vi "Jog.vi"(0 "AXIS Array":i32[](array[numeric]), 1 "U":bool, 2 "D":bool, 3 "R":bool, 4 "L":bool, 6 "Jog_Speed":i32=10000, 7 "Jog_相對位置":dbl format="%.2f", 9 "相對位置移動":bool, 10 "Jog Ring":u16(ring) items=["Step", "Continuous"], 11 "Step Ring":u16(ring) items=["0.001 mm", "0.01 mm", "0.1 mm", "1 mm"]) -> ()   [LabVIEW 2015]
uses:
  <userlib>/ADLINK/APS168.lvlib
panel:
  in  "角度逆轉":bool
  in  "角度正轉":bool
  in  "正轉":bool
  in  "逆轉":bool
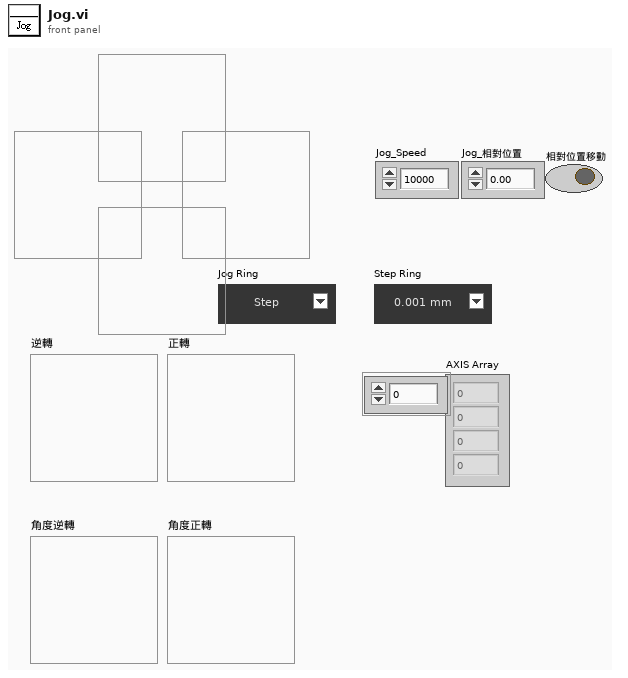
[diagram p1: front panel]
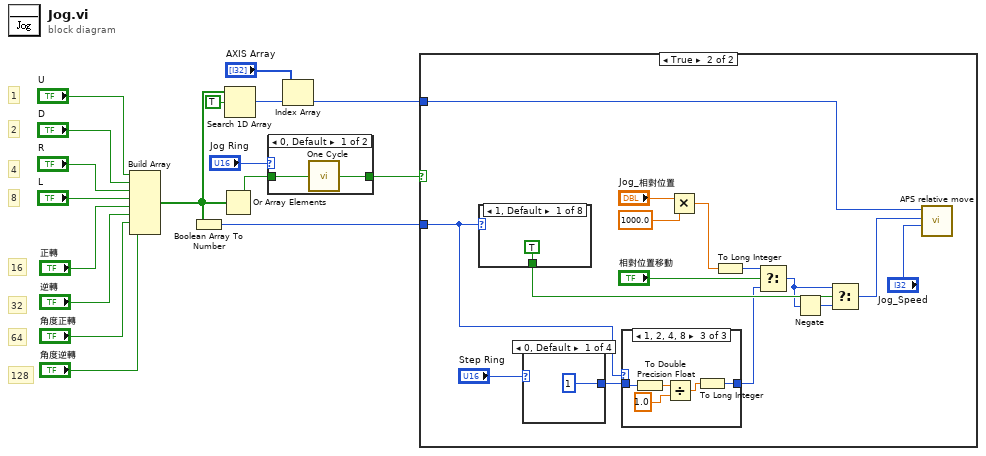
[diagram p0: block diagram]
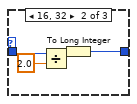
[diagram p5: hidden frame]
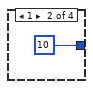
[diagram p6: hidden frame]
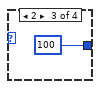
[diagram p7: hidden frame]
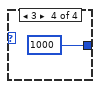
[diagram p8: hidden frame]
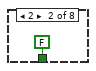
[diagram p9: hidden frame]
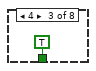
[diagram p10: hidden frame]
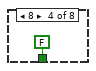
[diagram p11: hidden frame]
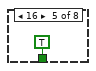
[diagram p12: hidden frame]
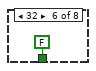
[diagram p13: hidden frame]
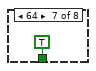
[diagram p14: hidden frame]
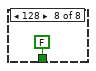
[diagram p15: hidden frame]
diagram:
  # "128"
  # "64"
  # "32"
  # "16"
  # "8"
  # "4"
  # "2"
  # "1"
  n1 = Build Array("U", "D", "R", "L", "正轉", "逆轉", "角度正轉", "角度逆轉") -> (w9:bool[])
  n2 = Boolean Array To Number(Boolean array=w9) -> (number=w17:u32)
  n3 = Or Array Elements(Boolean array=w9) -> (logical OR=w15:bool)
  n4 = Search 1D Array(1D array=w9, element=TRUE) -> (index of element=w7:i32)  [unwired: 1 in]
  n5 = case shown="0, Default" "Jog Ring" {
    tunnel: w15 -> [w19 w20]
    tunnel: [w18 w20] -> w14
    frame 0, Default {
      n6 = call "One Cycle.vi"("In"=w19) -> ("Out"=w18:bool)
    }
    frame 1 {
    }
  }
  n7 = Index Array(array="AXIS Array", index=w7) -> (element=w5:i32)
  n8 = case shown="True" w14 {
    tunnel: w17 -> [_ w33]
    tunnel: w5 -> [_ w21]
    frame False {
    }
    frame True {
      n9 = case shown="1, Default" w33 {
        tunnel: [TRUE FALSE TRUE FALSE TRUE FALSE TRUE FALSE] -> w35
        frame 1, Default {
        }
        frame 2 {
        }
        frame 4 {
        }
        frame 8 {
        }
        frame 16 {
        }
        frame 32 {
        }
        frame 64 {
        }
        frame 128 {
        }
      }
      n10 = case shown="0, Default" "Step Ring" {
        tunnel: [1 ("y") 10 ("y") 100 ("y") 1000 ("y")] -> w32
        frame 0, Default {
        }
        frame 1 {
        }
        frame 2 {
        }
        frame 3 {
        }
      }
      n11 = case shown="1, 2, 4, 8" w33 {
        tunnel: [w36 w37 w42] -> w25
        tunnel: w32 -> [w36 w40 w45]
        frame 0, Default {
        }
        frame 16, 32 {
          n12 = Divide(x=w40, y=2.0) -> (x/y=w38:dbl)
          n13 = To Long Integer(number=w38) -> (32bit integer=w37:i32)
        }
        frame 1, 2, 4, 8 {
          n14 = To Double Precision Float(number=w45) -> (double precision float=w41:dbl)
          n15 = Divide(x=w41, y=1.0) -> (x/y=w43:dbl)
          n16 = To Long Integer(number=w43) -> (32bit integer=w42:i32)
        }
      }
      n17 = Multiply(x="Jog_相對位置", y=1000.0) -> (x*y=w23:dbl)
      n18 = To Long Integer(number=w23) -> (32bit integer=w28:i32)
      n19 = Select(t=w28, s="相對位置移動", f=w25) -> (s? t:f=w26:i32)
      n20 = Negate(x=w26) -> (-x=w31:i32)
      n21 = Select(t=w26, s=w35, f=w31) -> (s? t:f=w27:i32)
      n22 = call <userlib>:"APS relative move.vi"("Max_Speed"="Jog_Speed", "Distance"=w27, "Axis_ID"=w21) -> ()  [unwired: 7 in, 2 out]
    }
  }
